vi "Update Calibration Time.vi"(8 "error in":errorcluster, 10 "Update Sites":i32[](array[numeric]), 11 "Offset Data":T1(array[cluster])) -> (0 "error out":errorcluster, 3 "Offset Data Out":T1(array[cluster]))   [LabVIEW 2020, in "GUCalibration2.lvlib"]
uses:
  GUCalibration2.lvlib
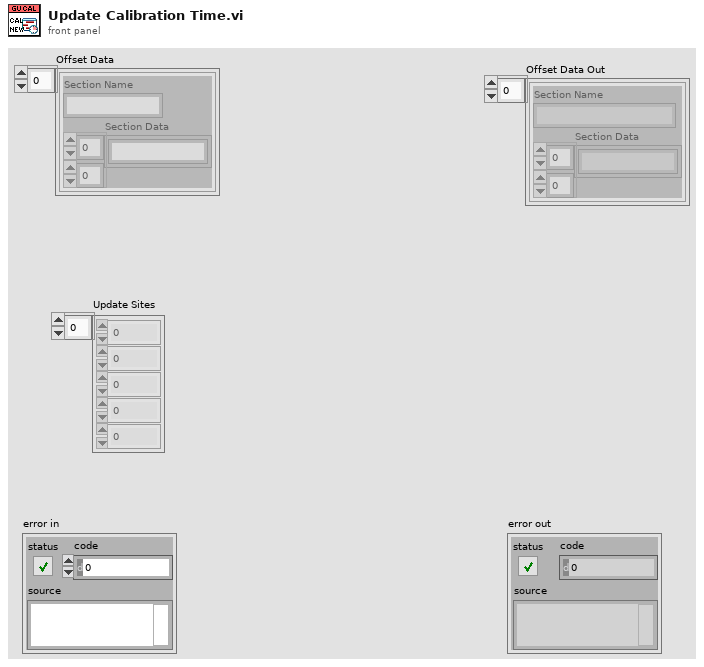
[diagram p1: front panel]
types:
  T1 = cluster{"Section Name":string, "Section Data":string[][]}[]
  T2 = cluster{"Section Name":string, "Section Data":string[][]}
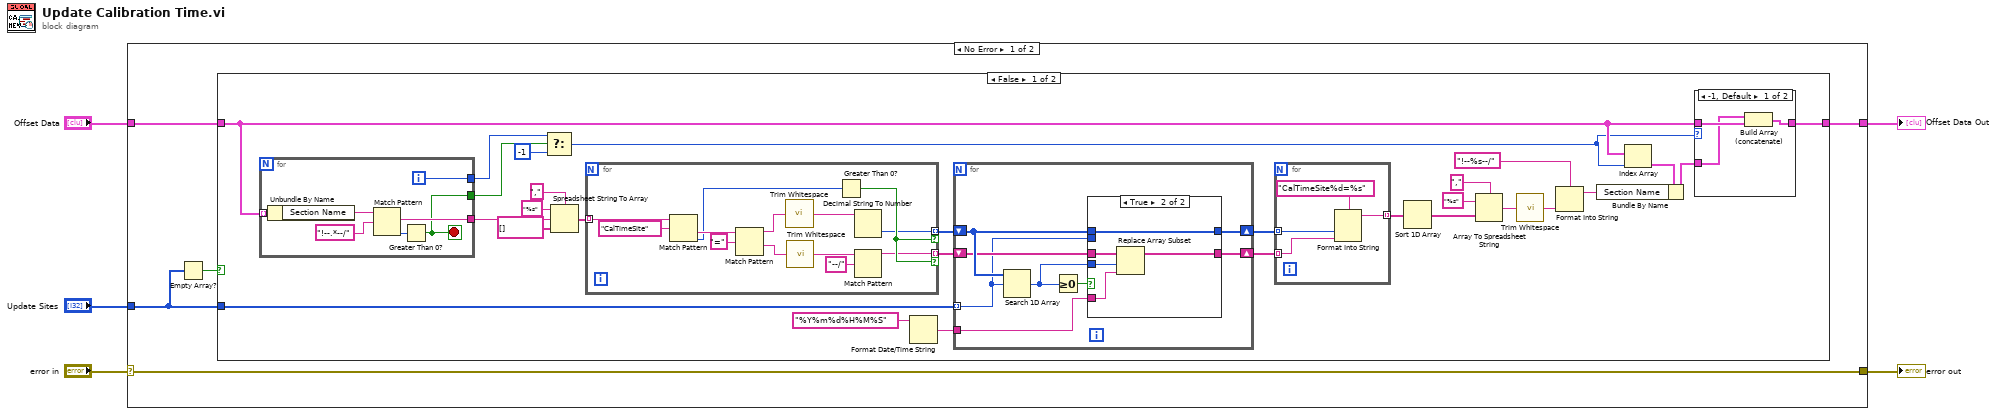
[diagram p0: block diagram]
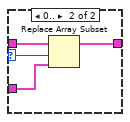
[diagram p2: hidden frame]
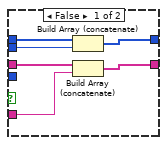
[diagram p3: hidden frame]
diagram:
  n1 = case shown="No Error" "error in" {
    selector: "error in" -> [w10 w91]
    tunnel: "Update Sites" -> [w7 _]
    tunnel: [w10 w91] -> w3
    tunnel: "Offset Data" -> [w9 w90]
    tunnel: [w8 w90] -> w2
    frame No Error {
      n2 = Empty Array?(array=w7) -> (empty?=w6:bool)
      n3 = case shown="False" w6 {
        tunnel: w7 -> [w32 _]
        tunnel: w9 -> [w19 w89]
        tunnel: [w17 w89] -> w8
        frame False {
          n4 = for {
            tunnel: w19 -> [w88] mode=indexing
            tunnel: [w84] -> w38
            tunnel: [w83] -> w15
            tunnel: [w82] -> w16
            i -> [w83]
            stop <- w82 stop-if-true
            n5 = Unbundle By Name(w88) -> ("Section Name"=w87:string)
            n6 = Match Pattern(string=w87, regular expression="!--.*--/") -> (match substring=w84:string, offset past match=w85:i32)  [unwired: 1 in, 2 out]
            n7 = Greater Than 0?(x=w85) -> (x > 0?=w82:bool)
          }
          n8 = Select(t=w15, s=w16, f=-1) -> (s? t:f=w13:i32)
          n9 = Spreadsheet String To Array(delimiter (Tab)=",", format string="%s", spreadsheet string=w38, array type (2D Dbl)=string[] []) -> (array=w34:string[])
          n10 = for {
            tunnel: w34 -> [w81] mode=indexing
            tunnel: [w72] -> w31 mode=indexing if=w74
            tunnel: [w69] -> w30 mode=indexing if=w74
            n11 = Match Pattern(string=w81, regular expression="CalTimeSite") -> (after substring=w79:string, offset past match=w75:i32)  [unwired: 1 in, 2 out]
            n12 = Match Pattern(string=w79, regular expression="=") -> (before substring=w77:string, after substring=w76:string)  [unwired: 1 in, 2 out]
            n13 = call <vilib>:"Trim Whitespace.vi"("string"=w77) -> ("trimmed string"=w73:string)  [unwired: 1 in]
            n14 = call <vilib>:"Trim Whitespace.vi"("string"=w76) -> ("trimmed string"=w71:string)  [unwired: 1 in]
            n15 = Greater Than 0?(x=w75) -> (x > 0?=w74:bool)
            n16 = Decimal String To Number(string=w73) -> (number=w72:i32)  [unwired: 2 in, 1 out]
            n17 = Match Pattern(string=w71, regular expression="--/") -> (before substring=w69:string)  [unwired: 1 in, 3 out]
          }
          n18 = Format Date/Time String(time format string (%c)="%Y%m%d%H%M%S") -> (date/time string=w29:string)  [unwired: 2 in]
          n19 = for {
            tunnel: w32 -> [w50] mode=indexing
            tunnel: w29 -> [w54]
            shift-right: [w53] -> w28
            shift-left: w31 -> [w56]
            shift-right: [w52] -> w27
            shift-left: w30 -> [w55]
            n20 = Search 1D Array(1D array=w56, element=w50) -> (index of element=w51:i32)  [unwired: 1 in]
            n21 = Greater Or Equal To 0?(x=w51) -> (x >= 0?=w57:bool)
            n22 = case shown="True" w57 {
              tunnel: w56 -> [w63 w67]
              tunnel: w55 -> [w61 w68]
              tunnel: w54 -> [w60 w66]
              tunnel: [w62 w67] -> w53
              tunnel: w51 -> [_ w65]
              tunnel: [w59 w64] -> w52
              tunnel: w50 -> [w58 _]
              frame False {
                n23 = Build Array (concatenate)(w63, w58) -> (w62:i32[])
                n24 = Build Array (concatenate)(w61, w60) -> (w59:string[])
              }
              frame True {
                n25 = Replace Array Subset(array=w68, new element=w66, index=w65) -> (w64:string[])
              }
            }
          }
          n26 = for {
            tunnel: w28 -> [w48] mode=indexing
            tunnel: w27 -> [w47] mode=indexing
            tunnel: [w46] -> w12 mode=indexing
            n27 = Format Into String(format string="CalTimeSite%d=%s" ("regular expression"), w48, w47) -> (resulting string=w46:string)  [unwired: 2 in, 1 out]
          }
          n28 = Sort 1D Array(array=w12) -> (sorted array=w11:string[])
          n29 = Array To Spreadsheet String(delimiter (Tab)=",", array=w11, 3:"%s" ("format string")) -> (spreadsheet string=w24:string)
          n30 = call <vilib>:"Trim Whitespace.vi"("string"=w24) -> ("trimmed string"=w23:string)  [unwired: 1 in]
          n31 = Format Into String(format string="!--%s--/", w23) -> (resulting string=w20:string)  [unwired: 2 in, 1 out]
          n32 = Index Array(array=w19, index=w13) -> (element=w21:T2)
          n33 = Bundle By Name(cluster=w21, "Section Name"=w20) -> (w18:T2)
          n34 = case shown="-1, Default" w13 {
            selector: w13 -> [_ w42]
            tunnel: w19 -> [w41 w45]
            tunnel: w18 -> [w39 w44]
            tunnel: [w40 w43] -> w17
            frame -1, Default {
              n35 = Build Array (concatenate)(w39, w41) -> (w40:T1)
            }
            frame 0.. {
              n36 = Replace Array Subset(array=w45, new element=w44, index=w42) -> (w43:T1)
            }
          }
        }
        frame True {
        }
      }
    }
    frame Error {
    }
  }
  "error out" <- w3
  "Offset Data Out" <- w2
